vi "A170316-11_IO.vi"() -> ()   [LabVIEW 2020]
uses:
  Libraries/S7/S7.lvlib
panel:
  in  "选项卡控件":enum32{"数字量输入", "数字量输出", "模拟量/伺服"}(tab)
  out "I 0":T1
  out "I 1":T2
  out "I 2":T3
  out "I 3":T4
  in  "Q 2":T5
  in  "Q 0":T6
  in  "Q 1":T7
  # "下轴装配"
  # "/"
  # "蜗杆伺服"
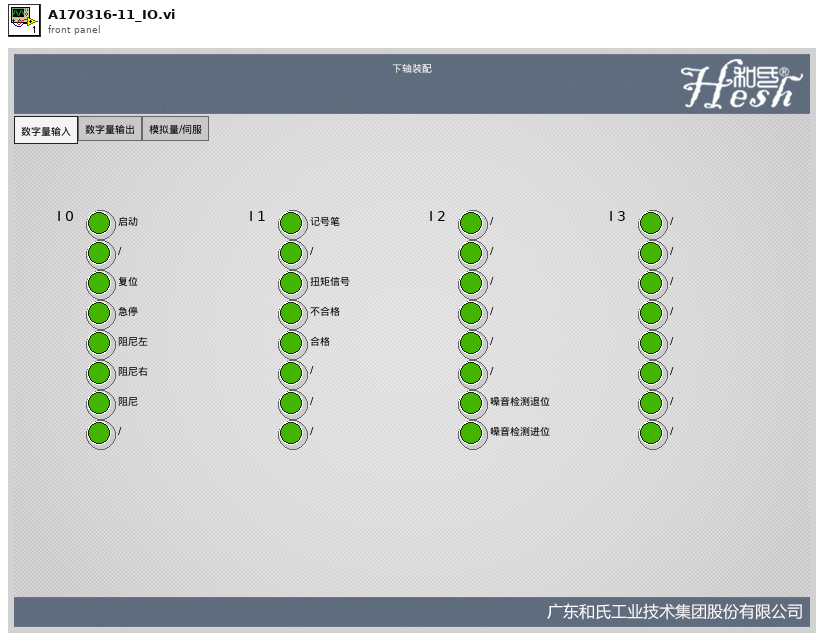
[diagram p1: front panel]
types:
  T1 = cluster{"启动":bool, "/":bool, "复位":bool, "急停":bool, "阻尼左":bool, "阻尼右":bool, "阻尼":bool, "/":bool}
  T2 = cluster{"记号笔":bool, "/":bool, "扭矩信号":bool, "不合格":bool, "合格":bool, "/":bool, "/":bool, "/":bool}
  T3 = cluster{"/":bool, "/":bool, "/":bool, "/":bool, "/":bool, "/":bool, "噪音检测退位":bool, "噪音检测进位":bool}
  T4 = cluster{"/":bool, "/":bool, "/":bool, "/":bool, "/":bool, "/":bool, "/":bool, "/":bool}
  T5 = cluster{bool, bool, "绿":bool, "黄":bool, "红":bool, "蜂鸣器":bool, "/":bool, "/":bool}
  T6 = cluster{bool, bool, bool, bool, "车速":bool, "点火":bool, "转速":bool, bool}
  T7 = cluster{"合格指示灯":bool, "不合格指示灯":bool, "噪音检测进":bool, "噪音检测退":bool, "/":bool, "/":bool, "/":bool, "/":bool}
  T8 = cluster{bool, bool, bool, bool, bool, bool, bool, bool}
  T9 = typedef "S7.lvlib/Read_Data (Reply Payload)--cluster.ctl" = cluster{"读取成功":bool, "数据":u32[], "Read_Data_error":errorcluster}
  T10 = cluster{"Boolean array[0]":bool, "Boolean array[1]":bool, "Boolean array[2]":bool, "Boolean array[3]":bool, "Boolean array[4]":bool, "Boolean array[5]":bool, "Boolean array[6]":bool, "Boolean array[7]":bool}
  T11 = cluster{"[0]":bool, "[1]":bool, "[2]":bool, "[3]":bool, "[4]":bool, "[5]":bool, "[6]":bool, "[7]":bool}
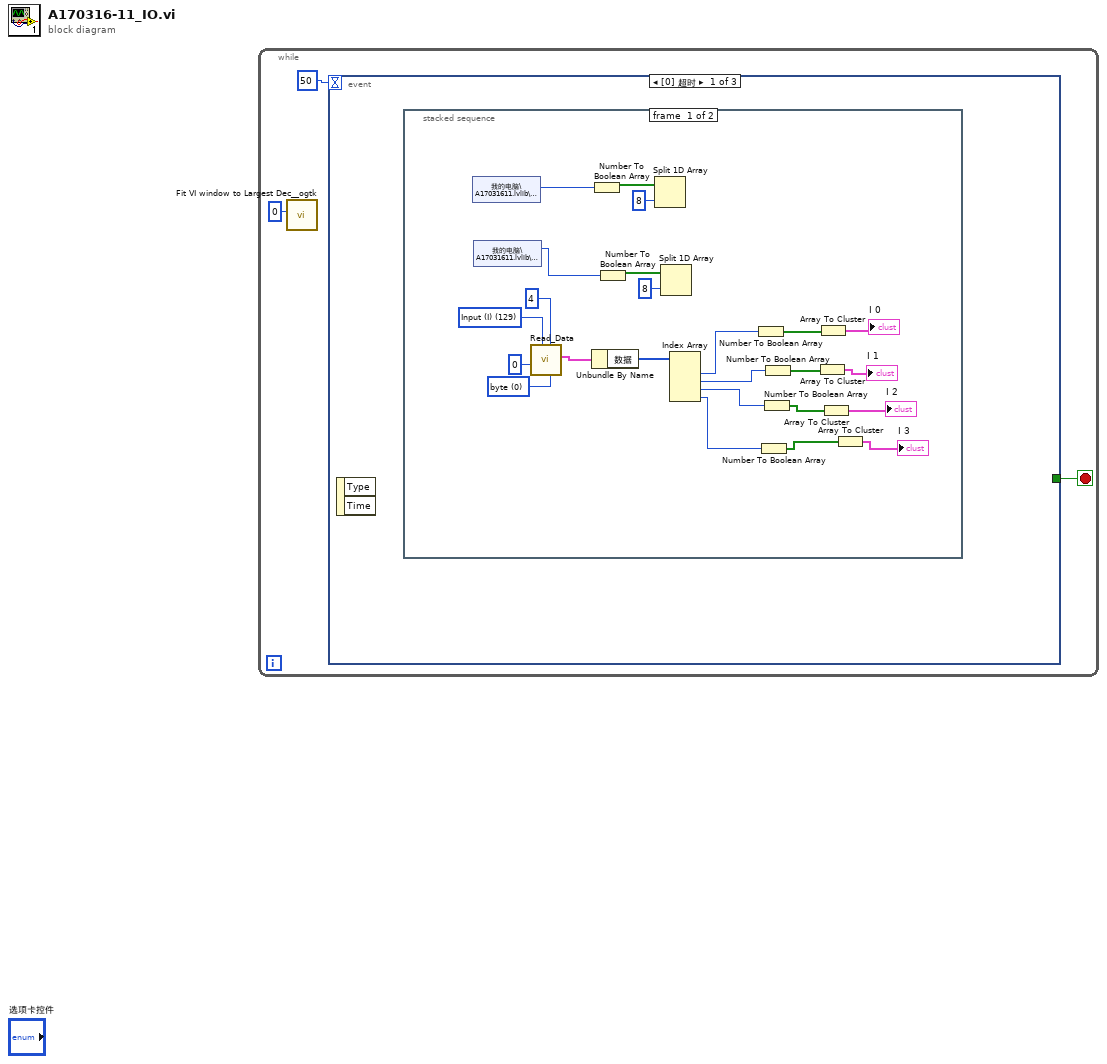
[diagram p0: block diagram]
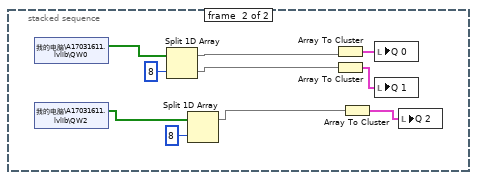
[diagram p2: hidden frame]
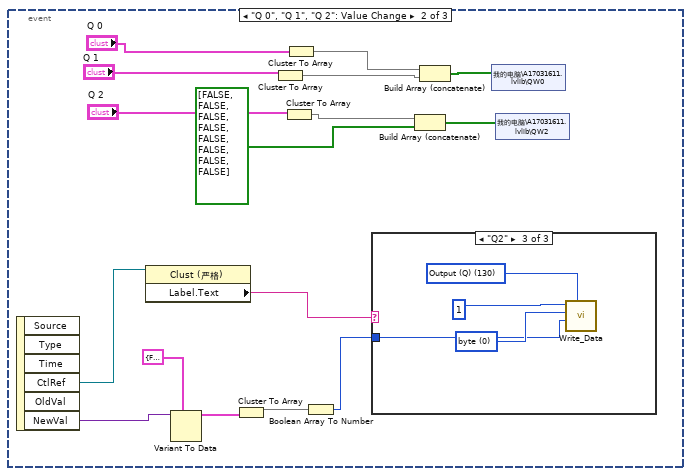
[diagram p3: hidden frame]
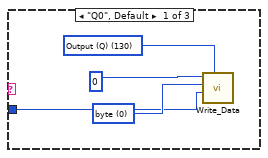
[diagram p4: hidden frame]
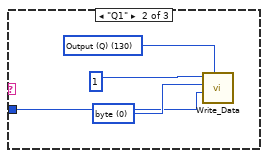
[diagram p5: hidden frame]
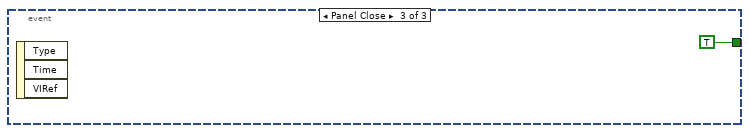
[diagram p6: hidden frame]
diagram:
  n1 = while {
    stop <- w3 stop-if-true
    n2 = call <userlib>:"Fit VI window to Largest Dec__ogtk.vi"("border spacing (2 px)"=0) -> ()  [unwired: 5 in, 2 out]
    n3 = event shown="[0] 超时" {
      selector: _ -> [_ _ _]
      dyn-events: _ -> [_ _ _]
      timeout: 50 -> [_ _ _]
      tunnel: [_ _ TRUE] -> w3
      event Timeout {
        n4 = event-data() -> ()  [unwired: 1 in, 2 out]
        n5 = stacked-sequence {
          frame #0 {
            w4 = u16 0 items=["byte", "word", "Dword"] ("数据类型")
            w17 = u8 129 items=["I/O (P)"=128, "Input (I)"=129, "Output (Q)"=130, "Bit Memory (M)"=131, "Data (DB)"=132, "Instance Data (DI)"=133, "Local Data (L)"=134, "Predecessor Local Data (VL)"=135] ("寄存器类型")
            n6 = shared-variable "我的电脑\\A17031611.lvlib\\IW0"() -> (w27:u16)  [unwired: 1 in, 1 out]
            n7 = shared-variable "我的电脑\\A17031611.lvlib\\IW2"() -> (w20:u16)  [unwired: 1 in, 1 out]
            n8 = call "Read_Data.vi"("数据类型"=w4, "读取长度"=u16 4, "寄存器类型"=w17, "起始地址"=u32 0) -> ("Reply Payload"=w14:T9)  [unwired: 5 in, 2 out]
            n9 = Number To Boolean Array(number=w27) -> (Boolean array=w26:bool[])
            n10 = Unbundle By Name(w14) -> ("数据"=w13:u32[])
            n11 = Number To Boolean Array(number=w20) -> (Boolean array=w21:bool[])
            n12 = Split 1D Array(array=w26, index=8 ("索引")) -> ()  [unwired: 2 out]
            n13 = Split 1D Array(array=w21, index=8 ("索引")) -> ()  [unwired: 2 out]
            n14 = Index Array(array=w13) -> (element #1=w12:u32, element #2=w11:u32, element #3=w10:u32, element #4=w9:u32)  [unwired: 4 in]
            n15 = Number To Boolean Array(number=w12) -> (Boolean array=w8:bool[])
            n16 = Number To Boolean Array(number=w9) -> (Boolean array=w5:bool[])
            n17 = Number To Boolean Array(number=w10) -> (Boolean array=w6:bool[])
            n18 = Number To Boolean Array(number=w11) -> (Boolean array=w7:bool[])
            n19 = Array To Cluster(array=w7) -> (cluster=→"I 1":T10)
            n20 = Array To Cluster(array=w8) -> (cluster=→"I 0":T10)
            n21 = Array To Cluster(array=w6) -> (cluster=→"I 2":T10)
            n22 = Array To Cluster(array=w5) -> (cluster=→"I 3":T10)
          }
          frame #1 {
            n23 = shared-variable "我的电脑\\A17031611.lvlib\\QW0"() -> (w34:bool[])  [unwired: 1 in, 1 out]
            n24 = shared-variable "我的电脑\\A17031611.lvlib\\QW2"() -> (w29:bool[])  [unwired: 1 in, 1 out]
            n25 = Split 1D Array(array=w34, index=8 ("索引")) -> (first subarray=w33:bool[], second subarray=w32:bool[])
            n26 = Split 1D Array(array=w29, index=8 ("索引")) -> (first subarray=w28:bool[])  [unwired: 1 out]
            n27 = Array To Cluster(array=w33) -> (cluster=w37:T11)
            n28 = Array To Cluster(array=w32) -> (cluster=w36:T11)
            n29 = Array To Cluster(array=w28) -> (cluster=w35:T11)
            n30 = local write "Q 0"(w37) -> ()
            n31 = local write "Q 1"(w36) -> ()
            n32 = local write "Q 2"(w35) -> ()
          }
        }
      }
      event "Q 0", "Q 1", "Q 2": Value Change {
        n33 = event-data() -> ("CtlRef"=w53:refnum<vi>, "NewVal"=w52:variant)  [unwired: 1 in, 4 out]
        n34 = property class="Clust (严格)"(reference=w53) -> ("Label.Text"=w42:string)  [unwired: 1 in, 2 out]
        n35 = Variant To Data(type=T8 {FALSE, FALSE, FALSE, FALSE, FALSE, FALSE, FALSE, FALSE}, Variant=w52) -> (data=w40:T8)  [unwired: 1 in, 1 out]
        n36 = Cluster To Array(cluster=w40) -> (array=w39:bool[])
        n37 = Cluster To Array(cluster="Q 1") -> (array=w50:bool[])
        n38 = Cluster To Array(cluster="Q 2") -> (array=w45:bool[])
        n39 = Cluster To Array(cluster="Q 0") -> (array=w51:bool[])
        n40 = Boolean Array To Number(Boolean array=w39) -> (number=w38:u32)
        n41 = case shown="\"Q2\"" w42 {
          tunnel: w38 -> [w54 w58 w62]
          frame "Q0", Default {
            w55 = u16 0 items=["byte", "word", "Dword"] ("数据类型")
            w57 = u8 130 items=["I/O (P)"=128, "Input (I)"=129, "Output (Q)"=130, "Bit Memory (M)"=131, "Data (DB)"=132, "Instance Data (DI)"=133, "Local Data (L)"=134, "Predecessor Local Data (VL)"=135] ("寄存器类型")
            n42 = call "Write_Data.vi"("寄存器类型"=w57, "写入数据"=w54, "数据类型"=w55, "写入地址"=u32 0 ("起始地址")) -> ()  [unwired: 5 in, 3 out]
          }
          frame "Q1" {
            w59 = u16 0 items=["byte", "word", "Dword"] ("数据类型")
            w61 = u8 130 items=["I/O (P)"=128, "Input (I)"=129, "Output (Q)"=130, "Bit Memory (M)"=131, "Data (DB)"=132, "Instance Data (DI)"=133, "Local Data (L)"=134, "Predecessor Local Data (VL)"=135] ("寄存器类型")
            n43 = call "Write_Data.vi"("寄存器类型"=w61, "写入数据"=w58, "数据类型"=w59, "写入地址"=u32 1 ("起始地址")) -> ()  [unwired: 5 in, 3 out]
          }
          frame "Q2" {
            w63 = u16 0 items=["byte", "word", "Dword"] ("数据类型")
            w65 = u8 130 items=["I/O (P)"=128, "Input (I)"=129, "Output (Q)"=130, "Bit Memory (M)"=131, "Data (DB)"=132, "Instance Data (DI)"=133, "Local Data (L)"=134, "Predecessor Local Data (VL)"=135] ("寄存器类型")
            n44 = call "Write_Data.vi"("寄存器类型"=w65, "写入数据"=w62, "数据类型"=w63, "写入地址"=u32 1 ("起始地址")) -> ()  [unwired: 5 in, 3 out]
          }
        }
        n45 = Build Array (concatenate)(w45, bool[] [FALSE, FALSE, FALSE, FALSE, FALSE, FALSE, FALSE, FALSE] ("数组")) -> (w44:bool[])
        n46 = Build Array (concatenate)(w51, w50) -> (w47:bool[])
        n47 = shared-variable "我的电脑\\A17031611.lvlib\\QW0"(w47) -> ()  [unwired: 1 in, 1 out]
        n48 = shared-variable "我的电脑\\A17031611.lvlib\\QW2"(w44) -> ()  [unwired: 1 in, 1 out]
      }
      event Panel Close {
        n49 = event-data() -> ()  [unwired: 1 in, 3 out]
      }
    }
  }
